vi "Check Can Write.vi"(8 "error in (no error)":errorcluster, 11 "Config Element in":refnum<class "Config Element.lvclass">) -> (0 "error out":errorcluster, 3 "Config Element out":refnum<class "Config Element.lvclass">)   [LabVIEW 2023, in "CDM-Config.lvlib" / "Config Element.lvclass"]
uses:
  Config Element.lvclass
  Config Element.lvclass/Config Element.ctl
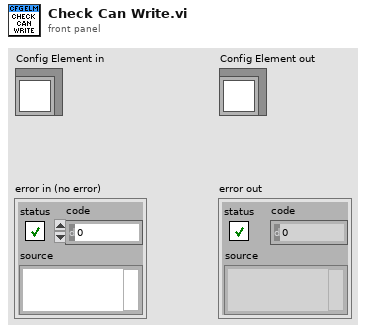
[diagram p1: front panel]
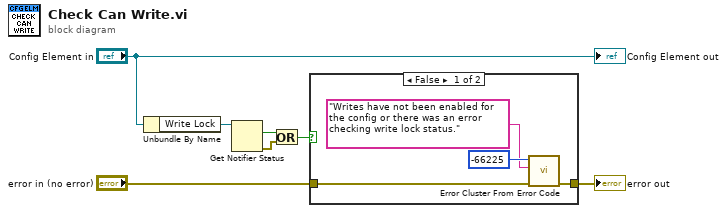
[diagram p0: block diagram]
diagram:
  n1 = Unbundle By Name("Config Element in") -> ("Write Lock"=w6:refnum<notifier>)
  n2 = Get Notifier Status(notifier=w6) -> (current notification=w5:bool, error out=w4:errorcluster)  [unwired: 1 in, 3 out]
  n3 = Or(x=w5, y=w4) -> (x .or. y?=w3:bool)
  n4 = case shown="False" w3 {
    tunnel: "error in (no error)" -> [w11 w12]
    tunnel: [w10 w12] -> w1
    frame False {
      n5 = call <vilib>:"Error Cluster From Error Code.vi"("error in (no error)"=w11, "error message (\"\")"="Writes have not been enabled for the config or there was an error checking write lock status.", "error code (0)"=-66225) -> ("error out"=w10:errorcluster)  [unwired: 6 in]
    }
    frame True {
    }
  }
  "error out" <- w1
  "Config Element out" <- "Config Element in"
